vi "MHL_forward file.vi"(0 "Delacor_lib_QMH_Message Queue in":refnum<class "Delacor_lib_QMH_Message Queue.lvclass">, 1 "Data Cluster in":T1, 5 "error in (no error)":errorcluster) -> (14 "Data Cluster out":T1, 19 "error out":errorcluster)   [LabVIEW 2019, in "Main UI.lvlib"]
uses:
  Main UI.lvlib
  <vilib>/Delacor/Delacor QMH/Libraries/Message Queue_class/Delacor_lib_QMH_Message Queue.lvclass
  Module Data--cluster.ctl
  Neo-Laura-LVOOP/Class Library/XYgraph_class/XYgraph.lvclass
  FileReader/FPref_clustered--cluster references.ctl
  Main UI Shared/Boolean--FP cluster.ctl
  FileReader/FPref_cntrls--cluster references.ctl
  Main UI Shared/Indicators--FP cluster.ctl
  <vilib>/Delacor/Delacor QMH/Libraries/Message Queue_class/Delacor_lib_QMH_Message Queue.lvclass/Delacor_lib_QMH_Message Queue.ctl
  <vilib>/Delacor/Delacor QMH/Libraries/Message Queue_class/Delacor_lib_QMH_Enqueue Message (Single).vi
  Main UI Shared/MAIN UI Shared.lvlib
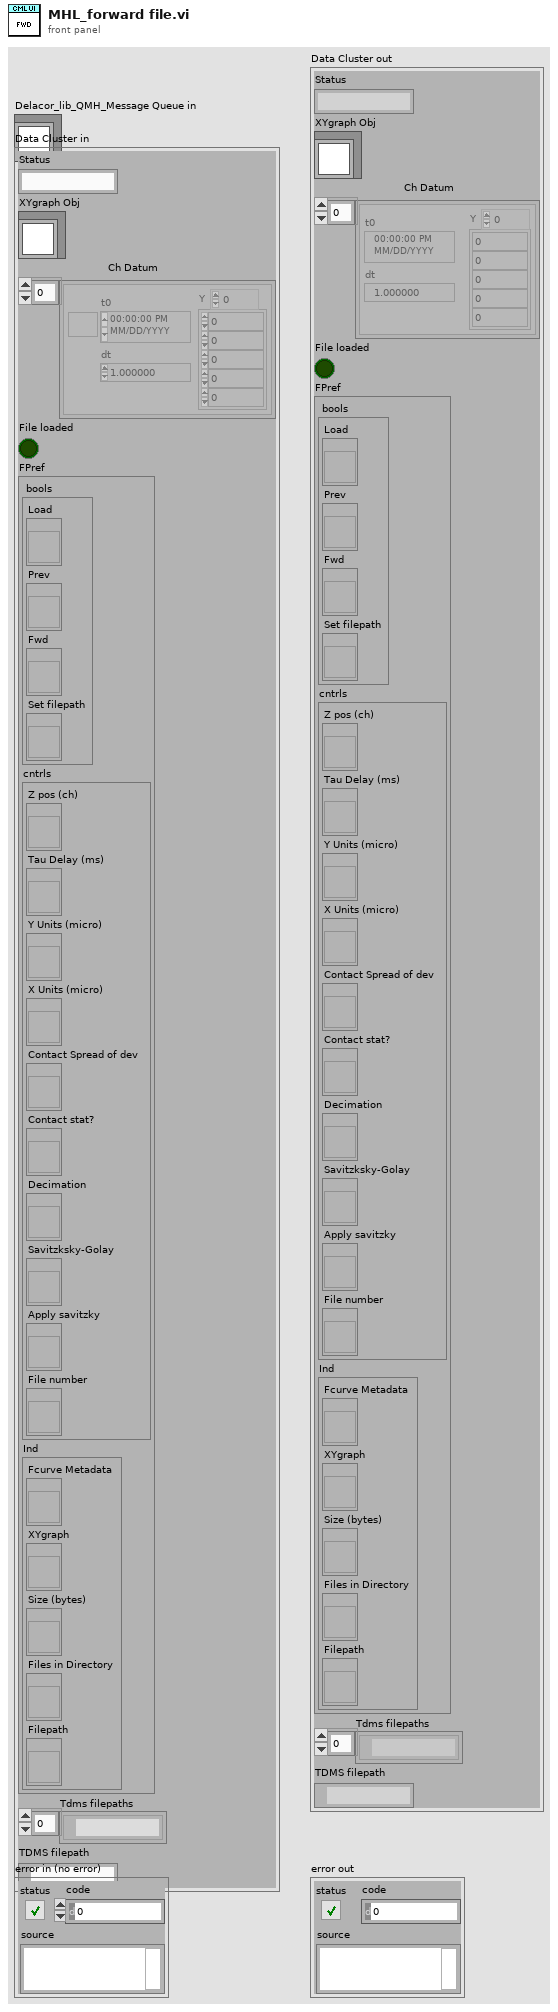
[diagram p1: front panel]
types:
  T1 = typedef "Main UI.lvlib/Module Data--cluster.ctl" = cluster{"Status":string, "XYgraph Obj":refnum<class "XYgraph.lvclass">, "Ch Datum":waveform(dbl)[], "File loaded":bool, "FPref":T2, "Tdms filepaths":path[], "TDMS filepath":path}
  T2 = typedef "FPref_clustered--cluster references.ctl" = cluster{" bools":T3, "cntrls":T4, "Ind":T5}
  T3 = typedef "MAIN UI Shared.lvlib/Boolean--FP cluster.ctl" = cluster{"Load":refnum<vi>, "Prev":refnum<vi>, "Fwd":refnum<vi>, "Set filepath":refnum<vi>}
  T4 = typedef "FPref_cntrls--cluster references.ctl" = cluster{"Z pos (ch)":refnum<vi>, "Tau Delay (ms)":refnum<vi>, "Y Units (micro)":refnum<vi>, "X Units (micro)":refnum<vi>, "Contact Spread of dev":refnum<vi>, "Contact stat?":refnum<vi>, "Decimation":refnum<vi>, "Savitzksky-Golay":refnum<vi>, "Apply savitzky ":refnum<vi>, "File number":refnum<vi>}
  T5 = typedef "Indicators--FP cluster.ctl" = cluster{"Fcurve Metadata":refnum<vi>, "XYgraph":refnum<vi>, "Size (bytes)":refnum<vi>, "Files in Directory":refnum<vi>, "Filepath":refnum<vi>}
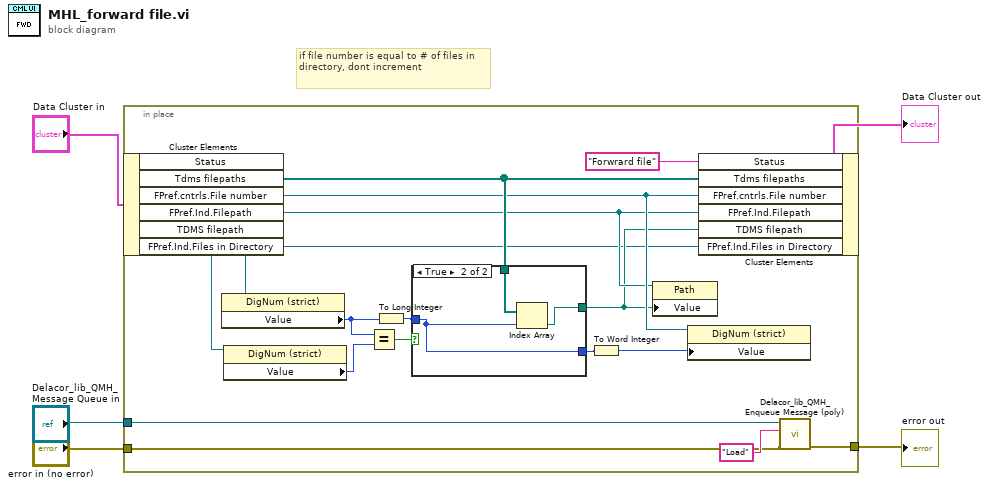
[diagram p0: block diagram]
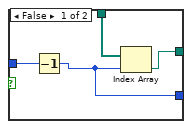
[diagram p2: hidden frame]
diagram:
  # "if file number is equal to # of files in directory, dont increment"
  n1 = in-place {
    in-place-border: "error in (no error)" -> [w20]
    in-place-border: [w19] -> w2
    in-place-border: "Delacor_lib_QMH_Message Queue in" -> [w17]
    n2 = in-place-cluster #1("Data Cluster in") -> ("Tdms filepaths"=w16:path[], "FPref.cntrls.File number"=w12:refnum<vi>, "FPref.Ind.Filepath"=w11:refnum<vi>, "FPref.Ind.Files in Directory"=w7:refnum<vi>)  [unwired: 2 out]
    n3 = property class="DigNum (strict)"(reference=w12) -> ("Value"=w15:i16)  [unwired: 1 in, 2 out]
    n4 = property class="DigNum (strict)"(reference=w7) -> ("Value"=w6:i16)  [unwired: 1 in, 2 out]
    n5 = Equal?(x=w15, y=w6) -> (x = y?=w14:bool)
    n6 = To Long Integer(number=w15) -> (32bit integer=w13:i32)
    n7 = case shown="True" w14 {
      tunnel: w16 -> [w25 w28]
      tunnel: w13 -> [w24 w26]
      tunnel: [w23 w26] -> w9
      tunnel: [w22 w27] -> w10
      frame False {
        n8 = Decrement(x=w24) -> (x-1=w23:i32)
        n9 = Index Array(array=w25, index=w23) -> (element=w22:path)
      }
      frame True {
        n10 = Index Array(array=w28, index=w26) -> (element=w27:path)
      }
    }
    n11 = To Word Integer(number=w9) -> (16bit integer=w8:i16)
    n12 = property class="Path"(reference=w11, "Value"=w10) -> ()  [unwired: 1 in, 2 out]
    n13 = property class="DigNum (strict)"(reference=w12, "Value"=w8) -> ()  [unwired: 1 in, 2 out]
    n14 = in-place-cluster #1("Status"="Forwrard file", "Tdms filepaths"=w16, "FPref.cntrls.File number"=w12, "FPref.Ind.Filepath"=w11, "TDMS filepath"=w10, "FPref.Ind.Files in Directory"=w7) -> (→"Data Cluster out":T1)
    n15 = call-poly <vilib>:"Delacor_lib_QMH_Enqueue Message (poly).vi"("error in"=w20, "Message"="Load", "Message Queue in"=w17) -> ("error out"=w19:errorcluster)  [unwired: 7 in, 1 out]
  }
  "error out" <- w2
